vi "Read_VN200.vi"(0 "FPGA Interface":refnum<k20>, 5 "error in":errorcluster) -> (4 "FPGA Interface Out":refnum<k20>, 6 "error out":errorcluster, 8 "Position Data":T1)   [LabVIEW 2016]
uses:
  Typedef/INS Data.ctl
  <vilib>/Utility/error.llb/Error Cluster From Error Code.vi
  <vilib>/rvi/errors/niLvFpgaAdjustHostInterfaceError.vi
  <vilib>/rvi/interface/nirviReadWriteControl/nirviReadWriteControl.xnode
  NiFpgaLv.dll
  <vilib>/rvi/interface/Simulation/niFpgaSimulationCallBeginRW.vi
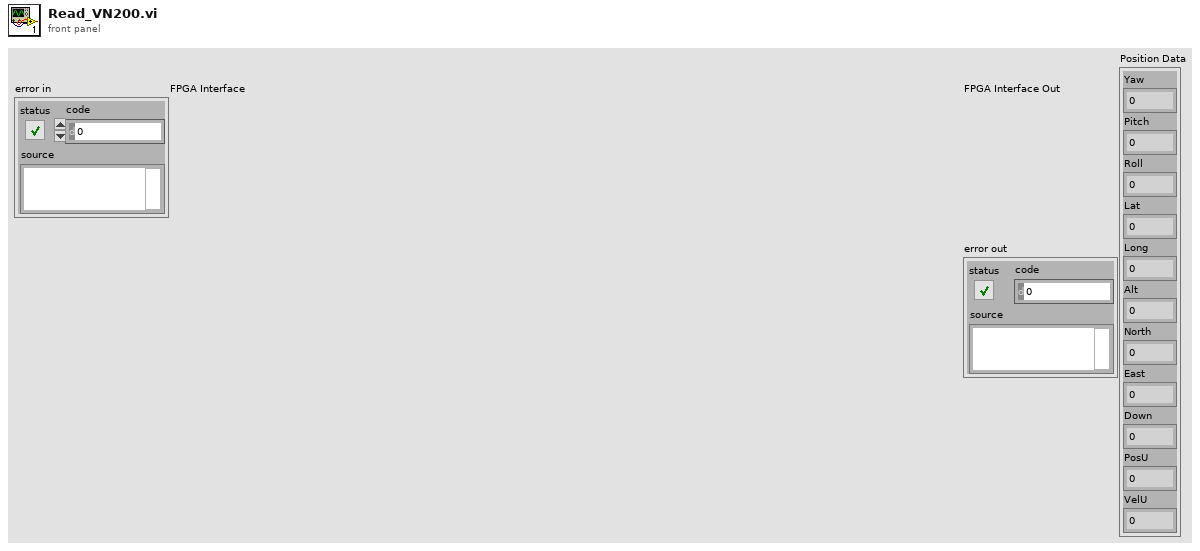
[diagram p1: front panel]
types:
  T1 = typedef "INS Data.ctl" = cluster{"Yaw":sgl, "Pitch":sgl, "Roll":sgl, "Lat":dbl, "Long":dbl, "Alt":dbl, "North":dbl, "East":dbl, "Down":dbl, "PosU":dbl, "VelU":dbl}
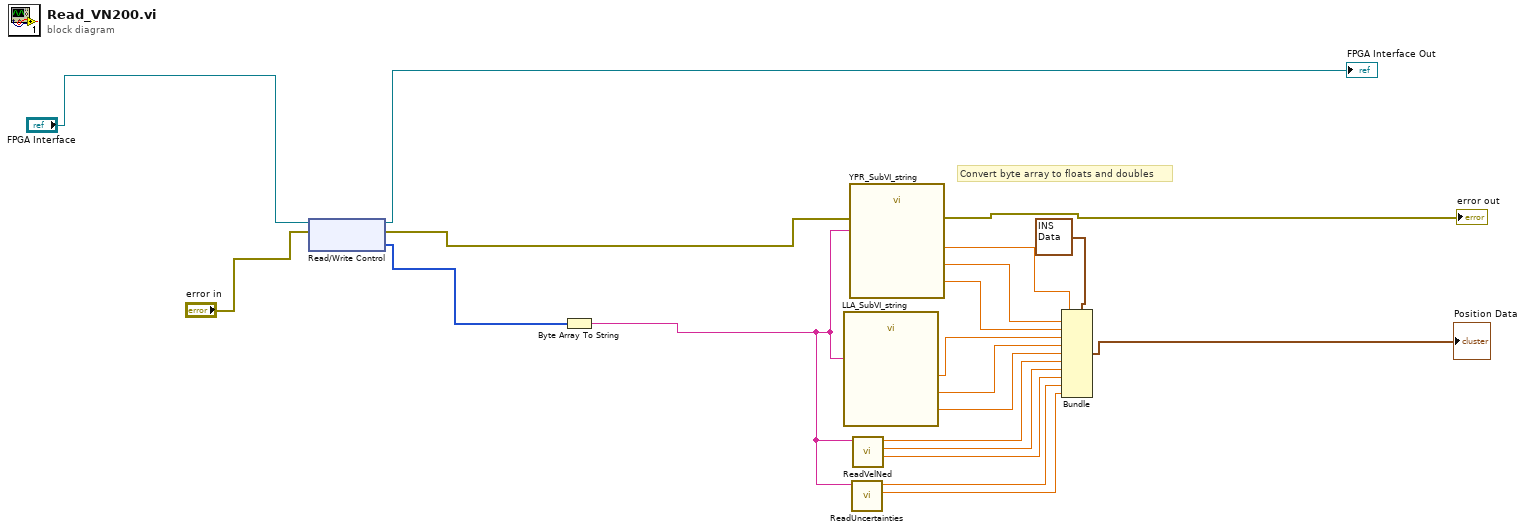
[diagram p0: block diagram]
diagram:
  # "Convert byte array to floats and doubles"
  n1 = xnode "Read/Write Control"("FPGA VI Reference In"="FPGA Interface", "error in"="error in") -> ("FPGA VI Reference Out"=→"FPGA Interface Out":refnum<k20>, "error out"=w15:errorcluster, "IMU_String"=w14:u8[])
  n2 = Byte Array To String(unsigned byte array=w14) -> (string=w16:string)
  n3 = call "LLA_SubVI_string.vi"("read buffer"=w16) -> ("Alt"=w8:dbl, "Long"=w9:dbl, "Lat"=w10:dbl)  [unwired: 8 in]
  n4 = call "YPR_SubVI_string.vi"("error in"=w15, "read buffer"=w16) -> ("error out"=→"error out":errorcluster, "Roll"=w11:sgl, "Pitch"=w12:sgl, "Yaw"=w13:sgl)  [unwired: 6 in]
  n5 = call "ReadUncertainties.vi"("read buffer"=w16) -> ("VelU"=w3:dbl, "PosU"=w4:dbl)  [unwired: 9 in]
  n6 = call "ReadVelNed.vi"("read buffer"=w16) -> ("Down"=w5:dbl, "East"=w6:dbl, "North"=w7:dbl)  [unwired: 8 in]
  n7 = Bundle(cluster=T1 {"Yaw"=0.0, "Pitch"=0.0, "Roll"=0.0, "Lat"=0.0, "Long"=0.0, "Alt"=0.0, "North"=0.0, "East"=0.0, "Down"=0.0, "PosU"=0.0, "VelU"=0.0} ("INS Data"), "Yaw"=w13, "Pitch"=w12, "Roll"=w11, "Lat"=w10, "Long"=w9, "Alt"=w8, "North"=w7, "East"=w6, "Down"=w5, "PosU"=w4, "VelU"=w3) -> (→"Position Data":T1)
